vi "File_FGV_sub_vi.vi"(8 "에러 입력":errorcluster, 9 "텍스트":string, 10 "열거형":enum16{"열기", "쓰기", "읽기", "닫기"}(ring), 11 "파일 경로(대화 상자 사용)":path) -> (0 "에러 출력":errorcluster, 2 "텍스트 2":string)   [LabVIEW 2020]
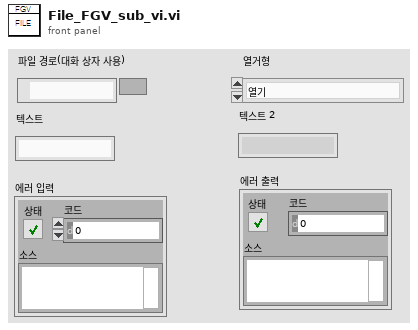
[diagram p1: front panel]
types:
  T1 = enum16{"open", "replace", "create", "open or create", "replace or create", "replace or create with confirmation"}
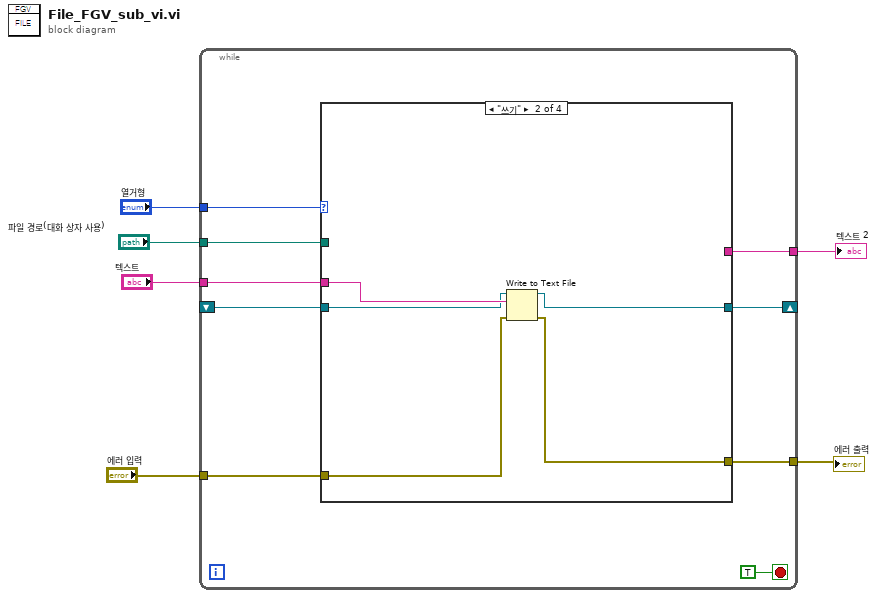
[diagram p0: block diagram]
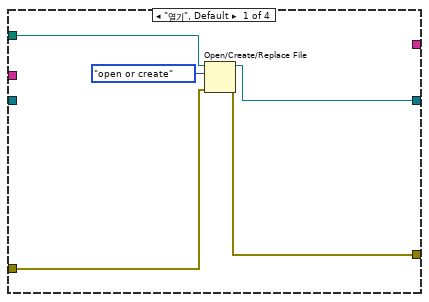
[diagram p2: hidden frame]
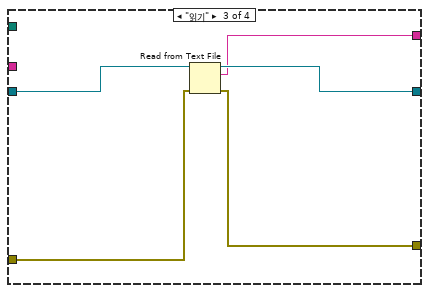
[diagram p3: hidden frame]
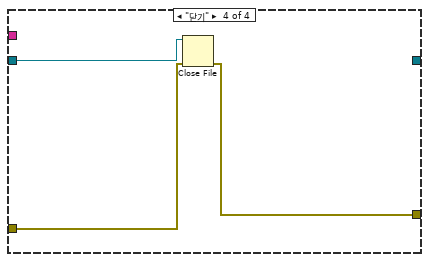
[diagram p4: hidden frame]
diagram:
  n1 = while {
    shift-right: [w11] -> _
    shift-left: _ -> [w7]
    tunnel: "열거형" -> [w14]
    tunnel: "파일 경로(대화 상자 사용)" -> [w13]
    tunnel: "에러 입력" -> [w12]
    tunnel: [w10] -> w3
    tunnel: "텍스트" -> [w9]
    tunnel: [w8] -> w1
    stop <- TRUE stop-if-true
    n2 = case shown="\"쓰기\"" w14 {
      tunnel: w13 -> [w19 _ _ _]
      tunnel: w12 -> [w18 w24 w29 w32]
      tunnel: [w17 w25 w28 _] -> w11
      tunnel: [w16 w23 w30 w31] -> w10
      tunnel: w9 -> [_ w22 _ _]
      tunnel: [_ _ w27 _] -> w8
      tunnel: w7 -> [_ w21 w26 w33]
      frame "열기", Default {
        n3 = Open/Create/Replace File(file path (use dialog)=w19, error in=w18, operation (0:open)=T1."open or create" ("동작(0:open)")) -> (refnum out=w17:refnum<file>, error out=w16:errorcluster)  [unwired: 3 in, 1 out]
      }
      frame "쓰기" {
        n4 = Write to Text File(file (use dialog)=w21, text=w22, error in=w24) -> (refnum out=w25:refnum<file>, error out=w23:errorcluster)  [unwired: 1 in, 1 out]
      }
      frame "읽기" {
        n5 = Read from Text File(file (use dialog)=w26, error in=w29) -> (refnum out=w28:refnum<file>, text=w27:string, error out=w30:errorcluster)  [unwired: 2 in, 1 out]
      }
      frame "닫기" {
        n6 = Close File(refnum=w33, error in=w32) -> (error out=w31:errorcluster)  [unwired: 1 out]
      }
    }
  }
  "에러 출력" <- w3
  "텍스트 2" <- w1
